vi "Fetch Device Info.vi"(8 "error in (no error)":errorcluster, 11 "PIC-Device in":refnum<class "PIC-Device.lvclass">) -> (0 "error out":errorcluster, 2 "Device Info":string[][](array[string]), 3 "PIC-Device out":refnum<class "PIC-Device.lvclass">)   [LabVIEW 2020, in "PIC-Device.lvclass"]
uses:
  PIC-Device.lvclass
  Toggle 8/Private/Get register for reading - array.vi
  Toggle 8/Toggle 8.lvclass
panel:
  out "class name":string
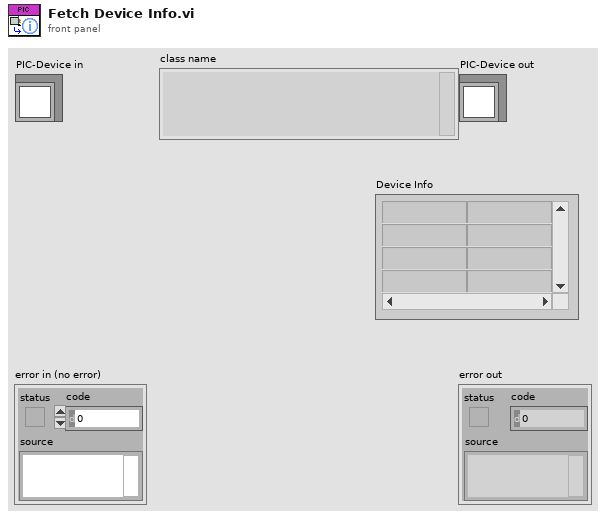
[diagram p1: front panel]
types:
  T1 = typedef "PIC-Device.lvclass/Register to Write.ctl" = cluster{"Register":u32, "Value":u32, "Dev Address":u32, "Physical Adress":u32}
  T2 = typedef "Device.lvclass/Device Information Cluster.ctl" = cluster{"Device Info":string[][], "Default Values":T1[], "Fetched info":string[][]}
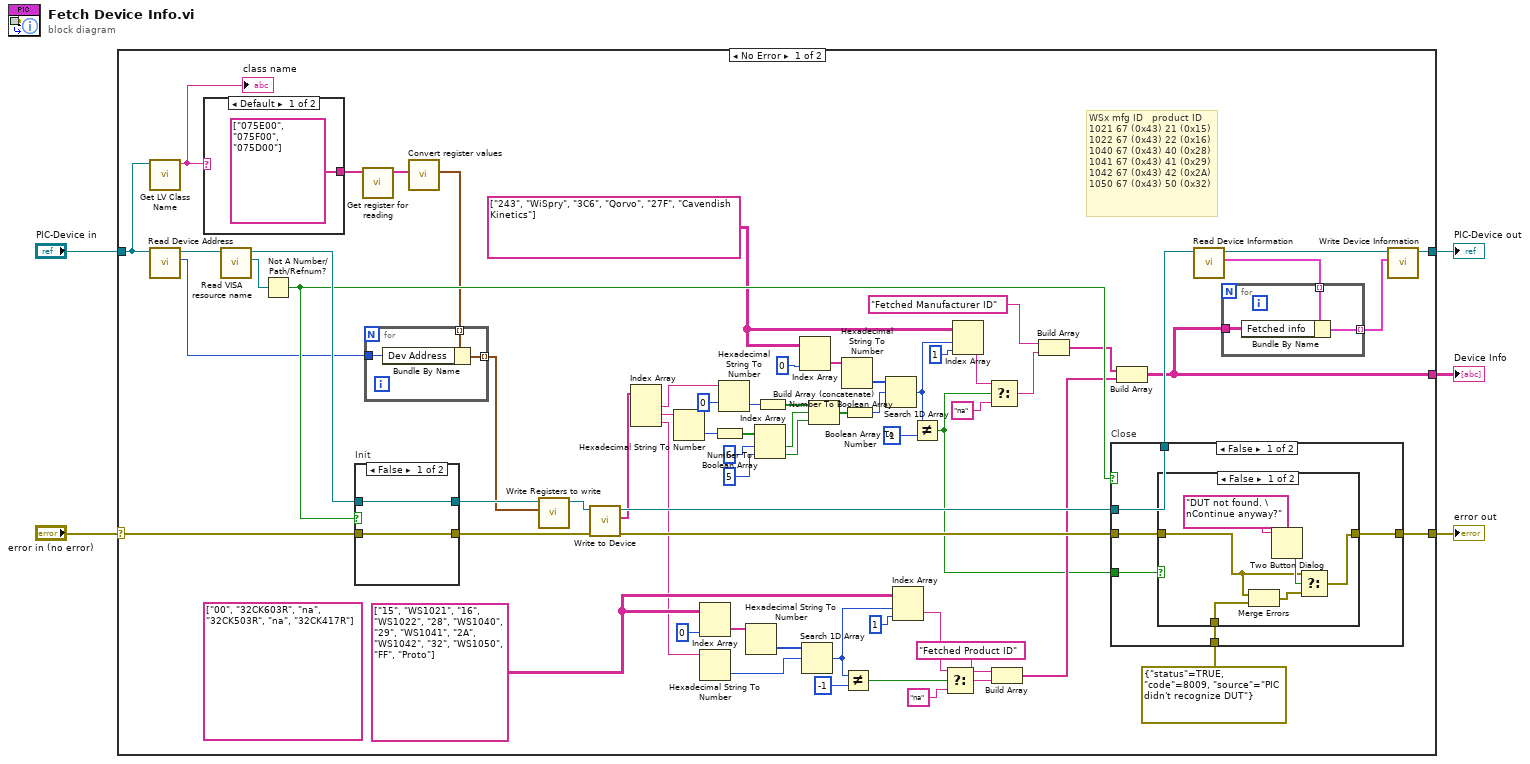
[diagram p0: block diagram]
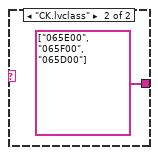
[diagram p2: hidden frame]
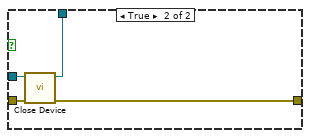
[diagram p4: hidden frame]
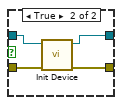
[diagram p5: hidden frame]
diagram:
  n1 = case shown="No Error" "error in (no error)" {
    selector: "error in (no error)" -> [w63 w104]
    tunnel: [w66 w104] -> w4
    tunnel: [w13 w103] -> w3
    tunnel: "PIC-Device in" -> [w21 w103]
    tunnel: [w12 _] -> w1
    frame No Error {
      (unwired) string[][] [["00", "32CK603R"], ["na", "32CK503R"], ["na", "32CK417R"]]
      w7 = string[][] [["243", "WiSpry"], ["3C6", "Qorvo"], ["27F", "Cavendish Kinetics"]]
      w32 = string[][] [["15", "WS1021"], ["16", "WS1022"], ["28", "WS1040"], ["29", "WS1041"], ["2A", "WS1042"], ["32", "WS1050"], ["FF", "Proto"]]
      # "WSx\tmfg ID \t\tproduct ID\n1021\t67 (0x43)\t21 (0x15)\n1022\t67 (0x43)\t22 (0x16)\n1040\t67 (0x43)\t40 (0x28)\n1041\t67 (0x43)\t41 (0x29)\n1042\t67 (0x43)\t42 (0x2A)\n1050\t67 (0x43)\t50 (0x32)"
      n2 = call <vilib>:"Get LV Class Name.vi"("object"=w21) -> ("class name"=w22:string)  [unwired: 9 in, 1 out]
      "class name" <- w22
      n3 = call-dynamic "Read Device Address.vi"("PIC-Device in"=w21) -> ("Device Address"=w18:u8, "PIC-Device out"=w20:refnum<class "PIC-Device.lvclass">)  [unwired: 9 in]
      n4 = case shown="Default" w22 {
        tunnel: [string[] ["075E00", "075F00", "075D00"] ("Reg array in") string[] ["065E00", "065F00", "065D00"] ("Reg array in")] -> w62
        frame Default {
        }
        frame "CK.lvclass" {
        }
      }
      n5 = call-dynamic "Read VISA resource name.vi"("Device in"=w20) -> ("VISA resource name"=w72:refnum<visa-resource-name>, "Device out"=w71:refnum<class "PIC-Device.lvclass">)  [unwired: 9 in]
      n6 = Not A Number/Path/Refnum?(number/path/refnum=w72) -> (NaN/Path/Refnum?=w61:bool)
      n7 = case "Init" shown="False" w61 {
        tunnel: w71 -> [w97 w102]
        tunnel: [w97 w101] -> w68
        tunnel: [w98 w100] -> w64
        tunnel: w63 -> [w98 w99]
        frame False {
        }
        frame True {
          n8 = call-dynamic "Init Device.vi"("error in (no error)"=w99, "Device in"=w102) -> ("error out"=w100:errorcluster, "Device out"=w101:refnum<class "PIC-Device.lvclass">)  [unwired: 8 in]
        }
      }
      n9 = call-poly "Get register for reading.vi"("Reg array in"=w62) -> ("Reg array out"=w69:string[])  [unwired: 10 in]
      n10 = call "Convert register values.vi"("Register strings"=w69) -> ("Register clusters out"=w19:T1[])  [unwired: 9 in, 1 out]
      n11 = for {
        tunnel: w19 -> [w78] mode=indexing
        tunnel: w18 -> [w77]
        tunnel: [w76] -> w17 mode=indexing
        n12 = Bundle By Name(cluster=w78, "Dev Address"=w77) -> (w76:T1)
      }
      n13 = call-dynamic "Write Registers to write.vi"("Registers to write"=w17, "Device in"=w68) -> ("Device out"=w70:refnum<class "PIC-Device.lvclass">)  [unwired: 9 in]
      n14 = call-dynamic "Write to Device.vi"("error in (no error)"=w64, "Device in"=w70) -> ("error out"=w65:errorcluster, "Return"=w43:string[], "Device out"=w67:refnum<class "PIC-Device.lvclass">)  [unwired: 7 in]
      n15 = Index Array(array=w43) -> (element #1=w41:string, element #2=w42:string, element #3=w28:string)  [unwired: 3 in]
      n16 = Hexadecimal String To Number(string=w42) -> (number=w60:u32)  [unwired: 2 in, 1 out]
      n17 = Index Array(array=w32, index (col)=0 ("disabled index (col)")) -> (element=w26:string[])  [unwired: 1 in]
      n18 = Hexadecimal String To Number(string=w28) -> (number=w27:u32)  [unwired: 2 in, 1 out]
      n19 = Number To Boolean Array(number=w60) -> (Boolean array=w54:bool[])
      n20 = Hexadecimal String To Number(string=w41, default (0uL)=u8 0 ("default (0 U32)")) -> (number=w23:u8)  [unwired: 1 in, 1 out]
      n21 = Hexadecimal String To Number(string=w26) -> (number=w25:u32[])  [unwired: 2 in, 1 out]
      n22 = Index Array(array=w54, index #1=6 ("index"), index #2=5 ("index")) -> (element #1=w56:bool, element #2=w55:bool)
      n23 = Number To Boolean Array(number=w23) -> (Boolean array=w57:bool[])
      n24 = Index Array(array=w7, index (col)=0 ("disabled index (col)")) -> (element=w53:string[])  [unwired: 1 in]
      n25 = Search 1D Array(1D array=w25, element=w27) -> (index of element=w38:i32)  [unwired: 1 in]
      n26 = Build Array (concatenate)(w57, w56, w55) -> (w24:bool[])
      n27 = Hexadecimal String To Number(string=w53) -> (number=w52:u32[])  [unwired: 2 in, 1 out]
      n28 = Not Equal?(x=w38, y=-1) -> (x != y?=w36:bool)
      n29 = Boolean Array To Number(Boolean array=w24) -> (number=w6:u32)
      n30 = Search 1D Array(1D array=w52, element=w6) -> (index of element=w49:i32)  [unwired: 1 in]
      n31 = Index Array(array=w32, index (row)=w38, index (col)=1 ("disabled index (col)")) -> (element=w35:string)
      n32 = Not Equal?(x=w49, y=-1) -> (x != y?=w10:bool)
      n33 = Select(t=w35, s=w36, f="na") -> (s? t:f=w33:string)
      n34 = Index Array(array=w7, index (row)=w49, index (col)=1 ("disabled index (col)")) -> (element=w47:string)
      n35 = Select(t=w47, s=w10, f="na") -> (s? t:f=w44:string)
      n36 = Build Array("Fetched Product ID" ("element"), w33) -> (w29:string[])
      n37 = Build Array("Fetched Manufacturer ID", w44) -> (w30:string[])
      n38 = case "Close" shown="False" w61 {
        tunnel: w67 -> [w85 w96]
        tunnel: [w85 w95] -> w14
        tunnel: [w82 w94] -> w66
        tunnel: w65 -> [w83 w93]
        tunnel: w10 -> [w84 _]
        tunnel: errorcluster {"status"=TRUE, "code"=8009, "source"="PIC didn't recognize DUT"} ("error out") -> [w81 _]
        frame False {
          n39 = case shown="False" w84 {
            tunnel: w83 -> [w88 w92]
            tunnel: [w86 w92] -> w82
            tunnel: w81 -> [w87 _]
            frame False {
              n40 = Merge Errors(w88, w87) -> (w89:errorcluster)
              n41 = Two Button Dialog(message="DUT not found. \nContinue anyway?") -> (T button?=w90:bool)  [unwired: 2 in]
              n42 = Select(t=w88, s=w90, f=w89) -> (s? t:f=w86:errorcluster)
            }
            frame True {
            }
          }
        }
        frame True {
          n43 = call-dynamic "Close Device.vi"("error in (no error)"=w93, "Device in"=w96) -> ("error out"=w94:errorcluster, "Device out"=w95:refnum<class "PIC-Device.lvclass">)  [unwired: 8 in]
        }
      }
      n44 = Build Array(w30, w29) -> (w12:string[][])
      n45 = call-dynamic "Read Device Information.vi"("Device in"=w14) -> ("Device Info"=w16:T2[], "Device out"=w11:refnum<class "PIC-Device.lvclass">)  [unwired: 8 in, 1 out]
      n46 = for {
        tunnel: w16 -> [w75] mode=indexing
        tunnel: w12 -> [w73]
        tunnel: [w74] -> w15 mode=indexing
        n47 = Bundle By Name(cluster=w75, "Fetched info"=w73) -> (w74:T2)
      }
      n48 = call-dynamic "Write Device Information.vi"("Device Info"=w15, "Device in"=w11) -> ("Device out"=w13:refnum<class "PIC-Device.lvclass">)  [unwired: 8 in, 1 out]
    }
    frame Error {
    }
  }
  "error out" <- w4
  "PIC-Device out" <- w3
  "Device Info" <- w1
